vi "Channel Topology Mapping Tester Tool.vi"() -> ()   [LabVIEW 2021]
uses:
  DMM SCAN DER/Typedefs/Scan Resource Names.ctl
  DMM SCAN DER/DMM_Scan DAQ Ext RLY.lvlib
panel:
  out "Topology Mapping Output":string[][](array[string])=[["ch0", "Voltage Type", "PXI_6363/port0/line0"], ["ch1", "Voltage Type", "PXI_6363/port0/line1"], ["ch2", "Voltage Type", "PXI_6363/port0/line2"], ["ch3", "Current Type ", "PXI_6363/port0/line3"], ["ch4", "Current Type ", "PXI_6363/port0/line4"], ["ch5", "Current Type ", "PXI_6363/port0/line5"], ["ch6", "Shunt Type linked to ch3", "PXI_6363/port0/line6"], ["ch7", "Shunt Type linked to ch4", "PXI_6363/port0/line7"], ["ch8", "Shunt Type linked to ch5", "PXI_6363/port0/line8"], ["ch9", "", "PXI_6363/port0/line9"], ["ch10", "", "PXI_6363/port0/line10"], ["ch11", "", "PXI_6363/port0/line11"], ["ch12", "", "PXI_6363/port0/line12"], ["ch13", "", "PXI_6363/port0/line13"], ["ch14", "", "PXI_6363/port0/line14"], ["ch15", "", "PXI_6363/port0/line15"], ["ch16", "", "PXI_6363/port0/line16"], ["ch17", "", "PXI_6363/port0/line17"], ["ch18", "", "PXI_6363/port0/line18"], ["ch19", "", "PXI_6363/port0/line19"], ["ch20", "", "PXI_6363/port0/line20"], ["ch21", "", "PXI_6363/port0/line21"], ["ch22", "", "PXI_6363/port0/line22"], ["ch23", "", "PXI_6363/port0/line23"], ["ch24", "", "PXI_6363/port0/line24"], ["ch25", "", "PXI_6363/port0/line25"], ["ch26", "", "PXI_6363/port0/line26"], ["ch27", "", "PXI_6363/port0/line27"], ["ch28", "", "PXI_6363/port0/line28"], ["ch29", "", "PXI_6363/port0/line29"], ["ch30", "", "PXI_6363/port0/line30"], ["ch31", "", "PXI_6363/port0/line31"], ["ch32", "", "PXI_6363/port1/line0"], ["ch33", "", "PXI_6363/port1/line1"], ["ch34", "", "PXI_6363/port1/line2"], ["ch35", "", "PXI_6363/port1/line3"], ["ch36", "", "PXI_6363/port1/line4"], ["ch37", "", "PXI_6363/port1/line5"], ["ch38", "", "PXI_6363/port1/line6"], ["ch39", "", "PXI_6363/port1/line7"], ["ch40", "", "PXI_6363/port2/line0"], ["ch41", "", "PXI_6363/port2/line1"], ["ch42", "", "PXI_6363/port2/line2"], ["ch43", "", "PXI_6363/port2/line3"], ["ch44", "", "PXI_6363/port2/line4"], ["ch45", "", "PXI_6363/port2/line5"], ["ch46", "", "PXI_6363/port2/line6"], ["ch47", "", "PXI_6363/port2/line7"]]
  in  "Channels Topology Mapping":T1={"Min Channel Voltage"=0, "Max Channel Voltage"=2, "Min Channel Current"=3, "Max Channel Current"=5, "N Shift Shunt to Min Channel Current"=3} caption="Channels Topology mapping"
  in  "Scan Resources Names":T2={"DMM Resource Name"="DMM_4065", "DAQ Resource Physical Channels Names"="PXI_6363/port0/line0:31, PXI_6363/port1/line0:7, PXI_6363/port2/line0:7"}
  out "error out":errorcluster
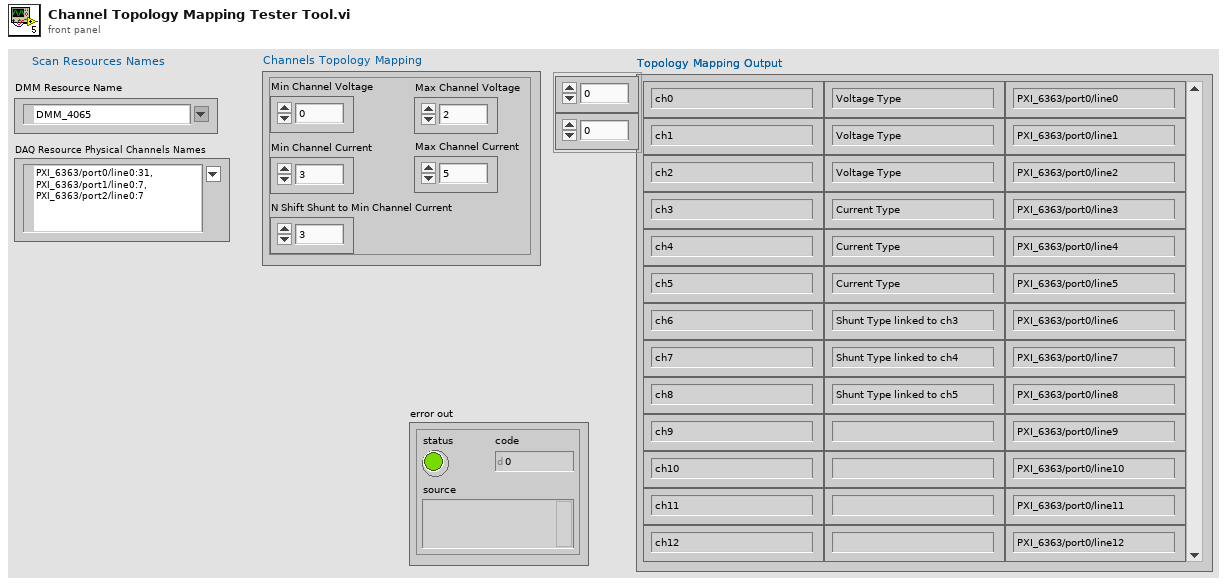
[diagram p1: front panel]
types:
  T1 = cluster{"Min Channel Voltage":u32, "Max Channel Voltage":u32, "Min Channel Current":u32, "Max Channel Current":u32, "N Shift Shunt to Min Channel Current":u32}
  T2 = typedef "DMM_Scan DAQ Ext RLY.lvlib/Scan Resource Names.ctl" = cluster{"DMM Resource Name":refnum<k15>, "DAQ Resource Physical Channels Names":tag}
  T3 = typedef "DMM_Scan DAQ Ext RLY.lvlib/Scan Resource Handles Out.ctl" = cluster{"DMM Handle":refnum<k15>, "DAQmx Task Out":refnum<k21>, "Relays Status Array":bool[], "N Shift Shunt":u32, "Close all Shunts?":bool, "Relays Debounce Time (ms)":u32}
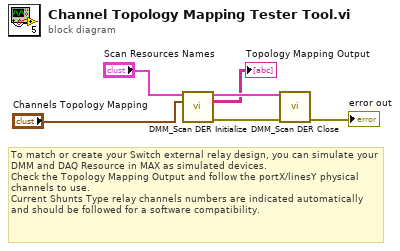
[diagram p0: block diagram]
diagram:
  # "To match or create your Switch external relay design, you can simulate your DMM and DAQ Resource in MAX as simulated devices.\nCheck the Topology Mapping Output and follow the portX/linesY physical channels to use.\nCurrent Shunts Type relay channels numbers are indicated automatically and should be followed for a software compatibility."
  n1 = call "DMM_Scan DER Initialize.vi"("Scan Resources Names"="Scan Resources Names", "Channels Topology Mapping"="Channels Topology Mapping") -> ("Scan Resources Handles Out"=w5:T3, "Topology Mapping Output"=→"Topology Mapping Output":string[][], "error out"=w6:errorcluster)  [unwired: 11 in]
  n2 = call "DMM_Scan DER Close.vi"("Scan Resources Handles In"=w5, "error in"=w6) -> ("error out"=→"error out":errorcluster)  [unwired: 13 in]
